vi "lv9_daqusb6251.vi"() -> ()   [LabVIEW 2009]
panel:
  out "Dinamômetro":string
  out "error out":errorcluster
  in  "VISA resource name":refnum<visa-resource-name>
  out "Final time [s]":dbl
  out "Iteration":i32
  out "Waveform Chart 2":dynamicdata(graph)
  in  "Device name":tag
  in  "Number of samples \nto read":i32
  in  "Acquisition rate [Hz]":dbl
  out "Waveform Chart":dynamicdata(graph)
  in  "Stop":bool
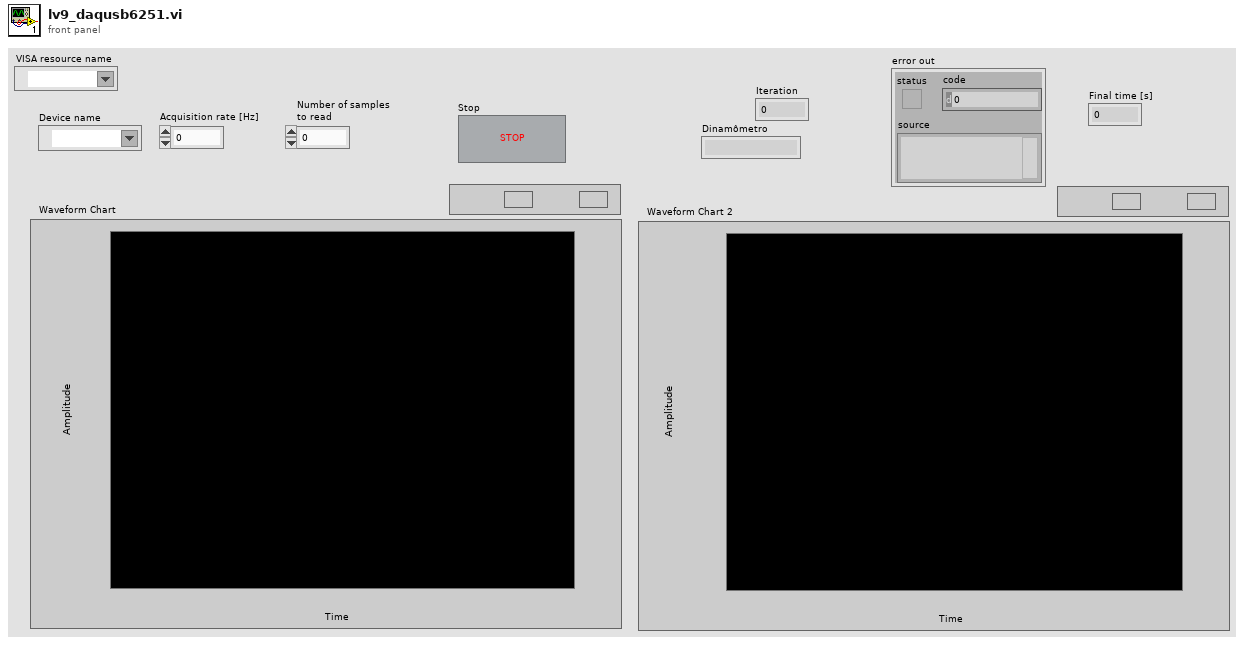
[diagram p1: front panel]
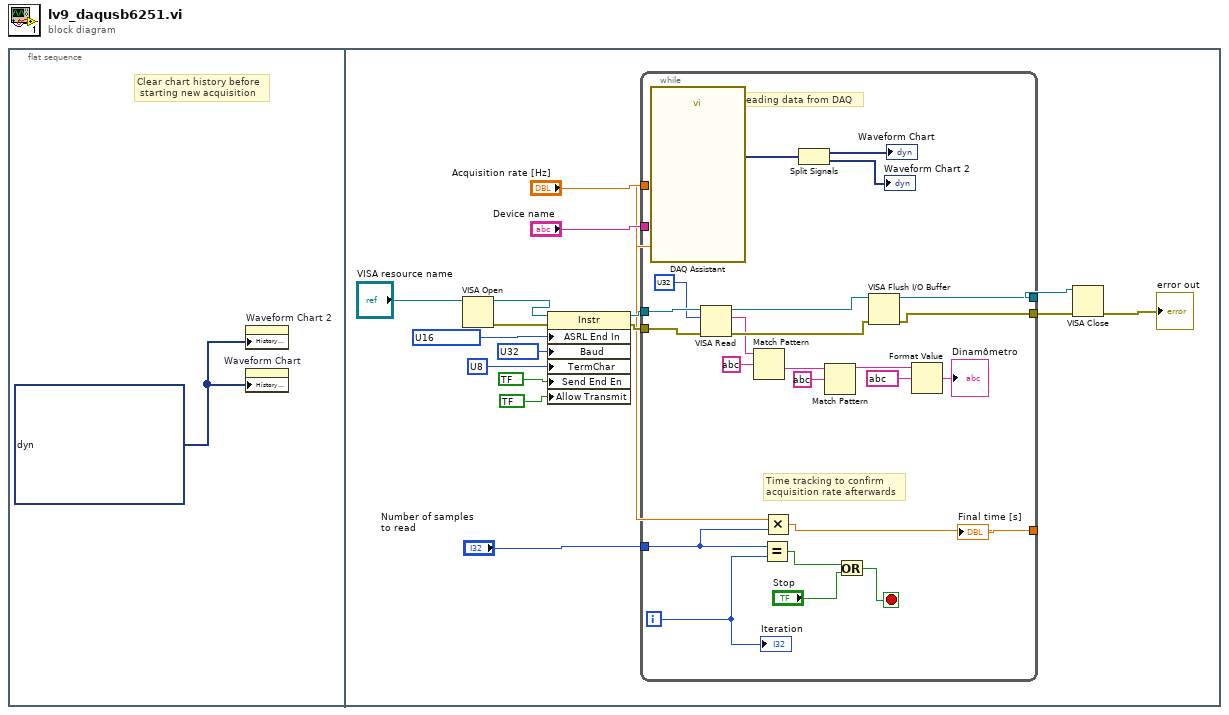
[diagram p0: block diagram]
diagram:
  n1 = flat-sequence {
    frame #0 {
      w1 = dynamicdata[] ? ("History Data")
      # "Clear chart history before\n starting new acquisition"
      n2 = property on="Waveform Chart 2" class="WFChart (strict)"("History Data"=w1) -> ()  [unwired: 2 in, 2 out]
      n3 = property on="Waveform Chart" class="WFChart (strict)"("History Data"=w1) -> ()  [unwired: 2 in, 2 out]
    }
    frame #1 {
      w4 = u16 ? items=["None", "Last Bit", "TermChar"] ("Serial Settings:End Mode for Reads")
      n4 = VISA Open(VISA resource name="VISA resource name") -> (VISA resource name=w7:refnum<visa-resource-name>, error out=w8:errorcluster)  [unwired: 4 in]
      n5 = property class="Instr"(reference=w7, error in=w8, "ASRL End In"=w4, "Baud"=u32 ? ("Serial Settings:Baud Rate"), "TermChar"=u8 ? ("Message Based Settings:Termination Character"), "Send End En"=bool ?, "Allow Transmit"=bool ?) -> (reference out=w10:refnum<visa-resource-name>, error out=w9:errorcluster)
      n6 = while {
        tunnel: "Device name" -> [_]
        tunnel: "Number of samples \nto read" -> [w36]
        tunnel: [w35] -> w17
        tunnel: "Acquisition rate [Hz]" -> [w34]
        tunnel: [w31] -> w14
        tunnel: [w29] -> w12
        tunnel: w10 -> [w28]
        tunnel: w9 -> [w27]
        i -> [w38]
        stop <- w39 stop-if-true
        # "Reading data from DAQ"
        # "Time tracking to confirm\nacquisition rate afterwards"
        n7 = call "DAQ Assistant"("rate"=w34) -> ("data"=w41:dynamicdata)  [unwired: 15 in, 3 out]
        n8 = VISA Read(VISA resource name=w28, byte count=u32 ?, error in (no error)=w27) -> (VISA resource name out=w32:refnum<visa-resource-name>, read buffer=w25:string, error out=w30:errorcluster)  [unwired: 1 out]
        n9 = Match Pattern(string=w25, regular expression=string ?) -> (after substring=w23:string)  [unwired: 1 in, 3 out]
        n10 = Equal?(x=w36, y=w38) -> (x = y?=w37:bool)
        n11 = Multiply(x=w34, y=w36) -> (x*y=w35:dbl)
        n12 = Split Signals(w41) -> (→"Waveform Chart":dynamicdata, →"Waveform Chart 2":dynamicdata)  [unwired: 2 in]
        n13 = Match Pattern(string=w23, regular expression=string ?) -> (before substring=w21:string)  [unwired: 1 in, 3 out]
        n14 = Or(x=w37, y="Stop") -> (x .or. y?=w39:bool)
        n15 = VISA Flush I/O Buffer(VISA resource name=w32, error in (no error)=w30) -> (VISA resource name out=w31:refnum<visa-resource-name>, error out=w29:errorcluster)  [unwired: 1 in]
        n16 = Format Value(string ("")=w21, format string=string ?) -> (output string=→"Dinamômetro":string)  [unwired: 1 in]
        "Iteration" <- w38
      }
      "Final time [s]" <- w17
      n17 = VISA Close(VISA resource name=w14, error in (no error)=w12) -> (error out=→"error out":errorcluster)
    }
  }
